vi "Setting Database.Refresh.vi"(8 "error in (no error)":errorcluster, 10 "Initialize":T1, 11 "Setting Database":refnum<class "Setting Database.lvclass">) -> (0 "error out":errorcluster, 3 "Setting Database out":refnum<class "Setting Database.lvclass">)   [LabVIEW 2019, in "Setting Database.lvclass"]
doc: "This will reset the list of Objects. This will set it to how many you specify in the input. If there are existing settings at an index, it will use those settings. If there is no existing settings, then it will use the default settings, which are accessed from an INI file in the default Lithography location. This will trigger the Settings Database to publish the following information: The new lists of Path, Rectangle and Funnel settings, as well as the new active objects (Funnel, Path, Rectangle etc). The active object index will also be returned to zero, so make sure that you handle the necessary UI changes."
uses:
  Setting Database.lvclass
  Typedefs/PrivateEvents--Setting Database.Refresh.ctl
  Setting Database.lvclass/Setting Database.ctl
panel:
  # "For instructions on how to use the JKI State Machine Objects, examples and video tutorials, visit:\nhttp://jki.net/state-machine-objects/\n\nJKI State Machine Objects™\nhttp://jki.net/state-machine-objects/\nCopyright (C) 2005-2015, JKI <info@jki.net>\nALL RIGHTS RESERVED"
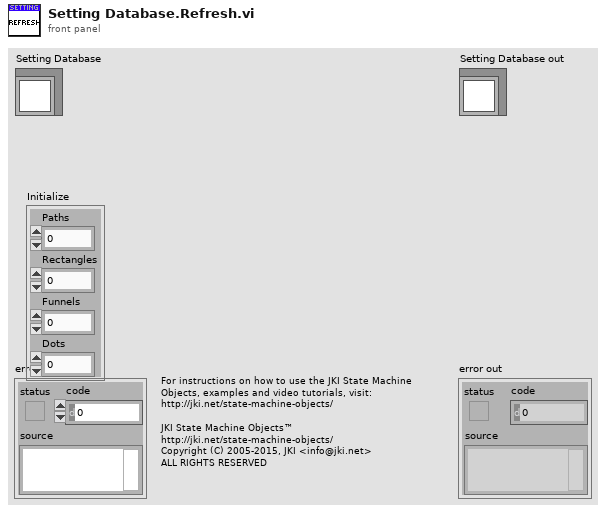
[diagram p1: front panel]
types:
  T1 = typedef "Setting Database.lvclass/PrivateEvents--Setting Database.Refresh.ctl" = cluster{"Paths":i32, "Rectangles":i32, "Funnels":i32, "Dots":i32}
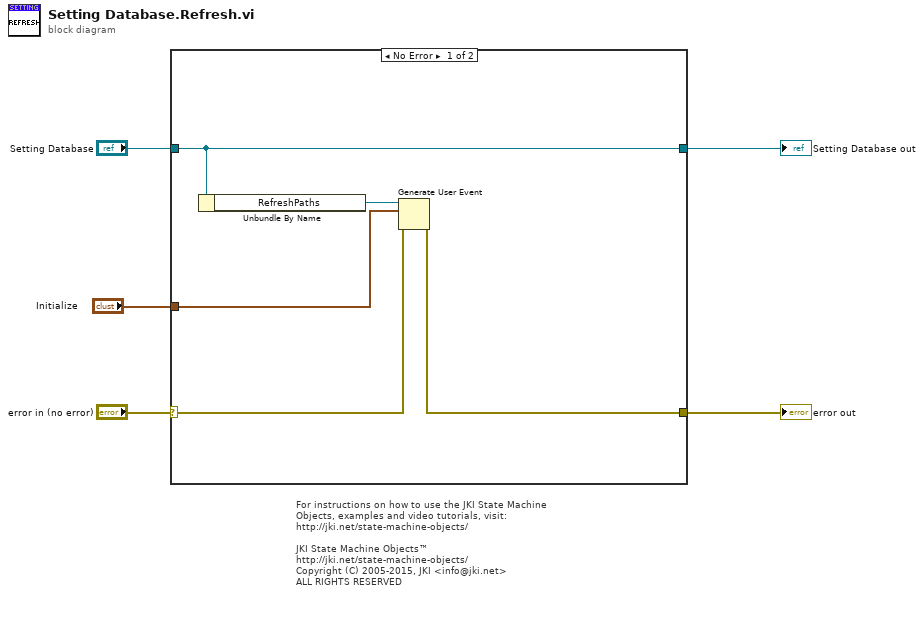
[diagram p0: block diagram]
diagram:
  # "For instructions on how to use the JKI State Machine Objects, examples and video tutorials, visit:\nhttp://jki.net/state-machine-objects/\n\nJKI State Machine Objects™\nhttp://jki.net/state-machine-objects/\nCopyright (C) 2005-2015, JKI <info@jki.net>\nALL RIGHTS RESERVED"
  n1 = case shown="No Error" "error in (no error)" {
    selector: "error in (no error)" -> [w10 w12]
    tunnel: [w7 w12] -> w4
    tunnel: [w6 w11] -> w5
    tunnel: "Setting Database" -> [w6 w11]
    tunnel: "Initialize" -> [w9 _]
    frame No Error {
      n2 = Unbundle By Name(w6) -> ("RefreshPaths"=w8:refnum<user-event>)
      n3 = Generate User Event(user event=w8, event data cluster=w9, error in=w10) -> (error out=w7:errorcluster)  [unwired: 1 in, 1 out]
    }
    frame Error {
    }
  }
  "error out" <- w4
  "Setting Database out" <- w5
